vi "Run.vi"(8 "error in (no error)":errorcluster, 9 "Type of Hexaboard":T1, 10 "Control In":T2={"I-O.lvclass"=refnum, "Gantry"=refnum, "Dispenser"="COM1"}, 11 "Assembly In":refnum<class "Database Assembly.lvclass">) -> (0 "error out":errorcluster, 2 "Control Out":T2={"I-O.lvclass"=refnum, "Gantry"=refnum, "Dispenser"="COM1"}, 3 "Assembly Out":refnum<class "Database Assembly.lvclass">)   [LabVIEW 2021, in "Database Assembly.lvclass"]
uses:
  Database Assembly.lvclass
  C:/Users/hep/Documents/UCSB-CMU-GantryCode/UCSB-Gantry-HEP-main (3)/UCSB-Gantry-HEP-main/Classes/Assembly/Assembly Run.lvclass
  Controller/Controllers.ctl
  Controller/I-O/I-O.lvclass
  C:/Program Files (x86)/Aerotech/A3200/LabVIEW/2010/Bin/Aerotech.A3200.dll
  Program Files (x86)/Aerotech/A3200/LabVIEW/2010/Bin/Aerotech.A3200.dll
  Routine/TypeOfHexaboard.ctl
  Database Assembly.lvclass/Database Assembly.ctl
  Assembly Run.lvclass
  Module/Module.lvclass
  Controller/Controller.lvclass
  Routine/Routine.lvclass
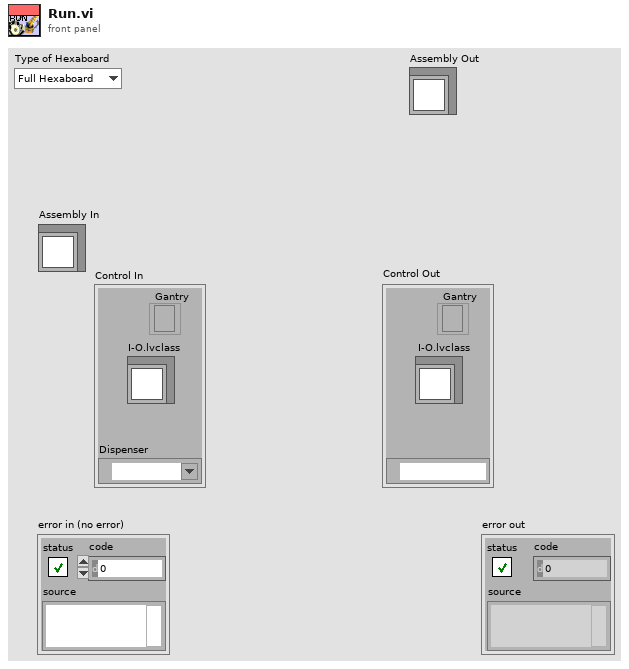
[diagram p1: front panel]
types:
  T1 = typedef "Routine.lvclass/TypeOfHexaboard.ctl" = enum16{"Full Hexaboard", "Right Partial PCB", "Right Partial Sensor", "Al Dummy Right Partial Sensor"}
  T2 = typedef "Controller.lvclass/Controllers.ctl" = cluster{"I-O.lvclass":refnum<class "I-O.lvclass">, "Gantry":refnum<k24>, "Dispenser":refnum<visa-resource-name>}
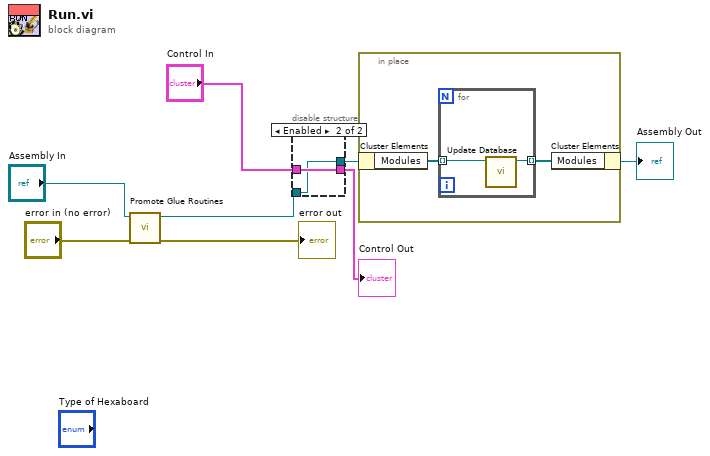
[diagram p0: block diagram]
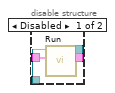
[diagram p2: hidden frame]
diagram:
  n1 = call "Promote Glue Routines.vi"("error in (no error)"="error in (no error)", "Assembly Run in"="Assembly In") -> ("error out"=→"error out":errorcluster, "Assembly Run out"=w4:refnum<class "Database Assembly.lvclass">)  [unwired: 8 in]
  n2 = disable-structure shown="Enabled" {
    disable-tunnel: w4 -> [w12 w13]
    disable-tunnel: [w11 w13] -> w3
    disable-tunnel: "Control In" -> [w10 w14]
    disable-tunnel: [w9 w14] -> w1
    frame Disabled {
      n3 = call-parent "Run.vi"("Control In"=w10, "Assembly In"=w12) -> ("Control Out"=w9:T2, "Assembly Out"=w11:refnum<class "Database Assembly.lvclass">)  [unwired: 7 in, 1 out]
    }
    frame Enabled {
    }
  }
  "Control Out" <- w1
  n4 = in-place {
    n5 = in-place-cluster #1(w3) -> ("Modules"=w16:refnum<class "Module.lvclass">[])
    n6 = for {
      tunnel: w16 -> [w18] mode=indexing
      tunnel: [w17] -> w15 mode=indexing
      n7 = call "Update Database.vi"("Module in"=w18) -> ("Module out"=w17:refnum<class "Module.lvclass">)  [unwired: 9 in, 1 out]
    }
    n8 = in-place-cluster #1("Modules"=w15) -> (→"Assembly Out":refnum<class "Database Assembly.lvclass">)
  }
